vi "test_SessionReservationInfo_ReserveSessions_SessionNamePrependedByInstrumentTypeId.vi"(8 "error in":errorcluster) -> (0 "error out":errorcluster, 2 "result":string, 3 "pass":bool)   [LabVIEW 2021, in "MeasurementServerTests.lvlib" / "Session Reservation Tests.lvlib"]
uses:
  Session Reservation Tests.lvlib
  gRPC/Generated APIs/ni/measurementlink/sessionmanagement/v1/RPC Messages/ni_measurementlink_PinMapContext.ctl
  Runtime/Clients/Session Management V1/Session Reservation/Session Reservation.lvclass/Session Reservation.ctl
  bff49ccc-0781-4f8a-a739-0c4a6493da00.vi
  c21ecf1c-8bb5-4f68-90ba-61375d462941.vi
  Runtime/Clients/Session Management V1/Session Reservation/Merge Invalid DVR Error.vi
  Helpers/Pin Map XML Strings Global.vi
  Runtime/Clients/Session Management V1/Session Reservation/Is DVR Valid.vi
  Runtime/Measurements/Helpers/Error Strings Global Internal.vi
  <vilib>/Utility/error.llb/Error Cluster From Error Code.vi
  <vilib>/JDP Science/JSONtext/Variant to JSON Text.vi
  <vilib>/JDP Science/JSONtext/LVClass Serializer/JSONtext LVClass Serializer.lvclass
  gRPC/Generated APIs/ni/measurementlink/sessionmanagement/v1/ni.measurementlink.sessionmanagement.v1.api.lvlib
  MeasurementServerTests.lvlib
  Runtime/Clients/Session Management V1/Session Reservation/Session Reservation.lvclass
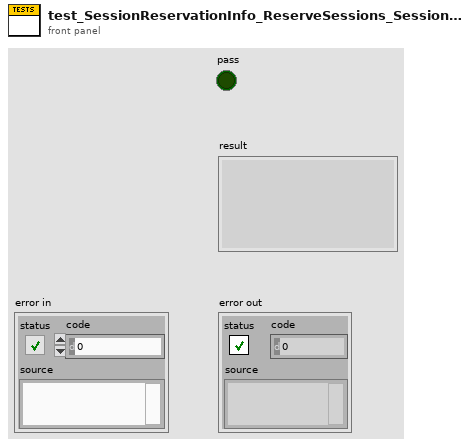
[diagram p1: front panel]
types:
  T1 = typedef "ni.measurementlink.sessionmanagement.v1.api.lvlib/ni_measurementlink_PinMapContext.ctl" = cluster{"pin_map_id":string, "sites":i32[]}
  T2 = typedef "ni.measurementlink.sessionmanagement.v1.api.lvlib/ni_measurementlink_sessionmanagement_v1_SessionInformation.ctl" = cluster{"session":T3, "resource_name":string, "channel_list":string, "instrument_type_id":string, "session_exists":bool, "session_reserved":bool, "channel_mappings":T4[], "annotations":T5[]}
  T3 = typedef "ni.measurementlink.sessionmanagement.v1.api.lvlib/nidevice_grpc_Session.ctl" = cluster{"name":string}
  T4 = typedef "ni.measurementlink.sessionmanagement.v1.api.lvlib/ni_measurementlink_sessionmanagement_v1_ChannelMapping.ctl" = cluster{"pin_or_relay_name":string, "site":i32, "channel":string, "multiplexer_resource_name":string, "multiplexer_route":string}
  T5 = typedef "ni.measurementlink.sessionmanagement.v1.api.lvlib/ni_measurementlink_sessionmanagement_v1_SessionInformation_AnnotationsEntry.ctl" = cluster{"key":string, "value":string}
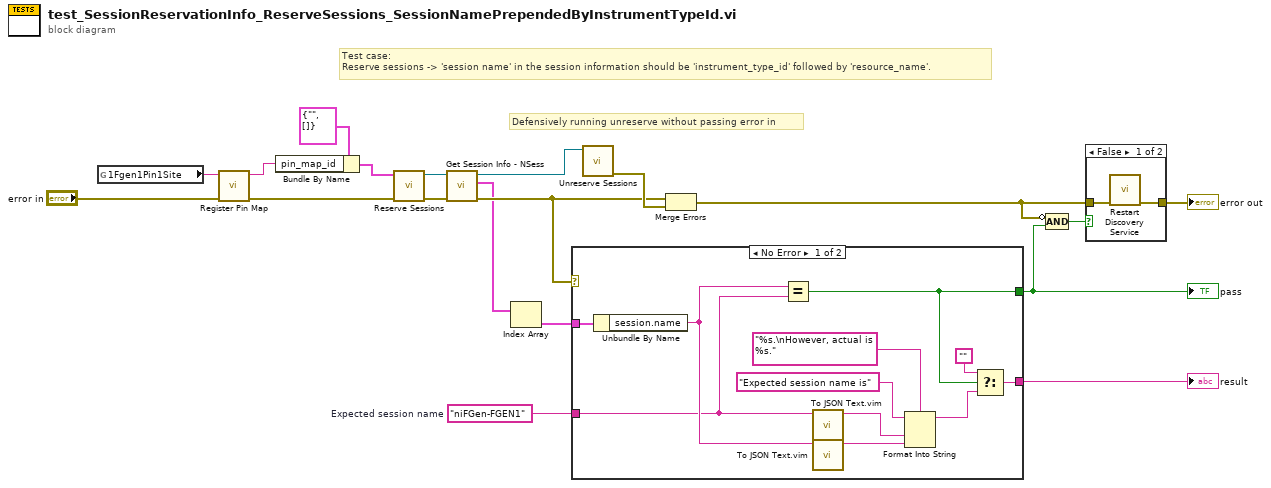
[diagram p0: block diagram]
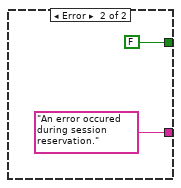
[diagram p3: hidden frame]
diagram:
  w2 = "niFGen-FGEN1"  # Expected session name
  # "Defensively running unreserve without passing error in"
  # "Test case:\nReserve sessions -> 'session name' in the session information should be 'instrument_type_id' followed by 'resource_name'."
  n1 = global read "Pin Map XML Strings Global.vi" "1Fgen1Pin1Site"() -> (w4:string)
  n2 = call "Register Pin Map.vi"("error in"="error in", "pin map xml"=w4) -> ("error out"=w15:errorcluster, "pin map id"=w16:string)  [unwired: 8 in]
  n3 = Bundle By Name(cluster=T1 {"pin_map_id"="", "sites"=[]} ("pin map context"), "pin_map_id"=w16) -> (w18:T1)
  n4 = call "Reserve Sessions.vi"("error in"=w15, "pin map context"=w18) -> ("error out"=w17:errorcluster, "session reservation out"=w7:refnum<class "Session Reservation.lvclass">)  [unwired: 8 in]
  n5 = call "Get Session Info - NSess .vi"("error in"=w17, "session reservation in"=w7) -> ("error out"=w9:errorcluster, "sessions info"=w1:T2[], "session reservation out"=w11:refnum<class "Session Reservation.lvclass">)  [unwired: 7 in]
  n6 = Index Array(array=w1) -> (element=w10:T2)  [unwired: 1 in]
  n7 = case shown="No Error" w9 {
    tunnel: [w21 FALSE] -> w6
    tunnel: [w26 "An error occured during session reservation." ("String")] -> w5
    tunnel: w10 -> [w22 _]
    tunnel: w2 -> [w20 _]
    frame No Error {
      n8 = Unbundle By Name(w22) -> ("session.name"=w24:string)
      n9 = Equal?(x=w24, y=w20) -> (x = y?=w21:bool)
      n10 = call "To JSON Text.vim"("Anything"=w20) -> ("<JSON>"=w23:string)  [unwired: 9 in, 1 out]
      n11 = call "To JSON Text.vim"("Anything"=w24) -> ("<JSON>"=w25:string)  [unwired: 9 in, 1 out]
      n12 = Format Into String(format string="%s.\nHowever, actual is %s.", initial string="Expected session name is", w23, w25) -> (resulting string=w29:string)  [unwired: 1 in, 1 out]
      n13 = Select(t="", s=w21, f=w29) -> (s? t:f=w26:string)
    }
    frame Error {
    }
  }
  "pass" <- w6
  "result" <- w5
  n14 = call "Unreserve Sessions.vi"("session reservation in"=w11) -> ("error out"=w12:errorcluster)  [unwired: 10 in]
  n15 = Merge Errors(w9, w12) -> (w13:errorcluster)
  n16 = Compound Arithmetic op=AND(invert w13, w6) -> (w14:bool)
  n17 = case shown="False" w14 {
    tunnel: [w34 w35] -> w8
    tunnel: w13 -> [w33 w35]
    frame False {
      n18 = call "Restart Discovery Service.vi"("error in"=w33) -> ("error out"=w34:errorcluster)  [unwired: 10 in]
    }
    frame True {
    }
  }
  "error out" <- w8
